vi "UpdateFilterMap.vi"(9 "MailBoxMessage":refnum<class "MailBoxMessage.lvclass">, 10 "_Msg-Filter":refnum<class "_Msg-Filter.lvclass">, 11 "MailboxClient in":refnum<class "MailboxClient.lvclass">) -> (3 "MailboxClient out":refnum<class "MailboxClient.lvclass">)   [LabVIEW 2020, in "MailboxClient.lvlib" / "MailboxClient.lvclass"]
uses:
  MailboxClient.lvclass
  <vilib>/Utility/miscctls.llb/LVMapReplaceAction.ctl
  MailboxManager/MailBoxMessage/MailBoxMessage.lvclass
  C:/Program Files (x86)/National Instruments/LabVIEW 2020/vi.lib/ActorFramework/Message/Message.lvclass
  C:/Users/taylo/Projects/LabVIEW/ActorMailbox/MailboxManager/MailBoxMessage/MailBoxMessage.lvclass
  MailboxManager/_Msg-Filter/_Msg-Filter.lvclass
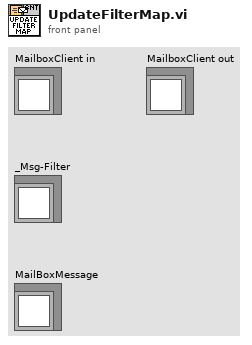
[diagram p1: front panel]
types:
  T1 = typedef "LVMapReplaceAction.ctl" = enum32{"Modify Entry only if found", "Add or Modify Entry", "Delete Entry"}
  T2 = map{refnum<class "Message.lvclass">, refnum<class "_Msg-Filter.lvclass">}
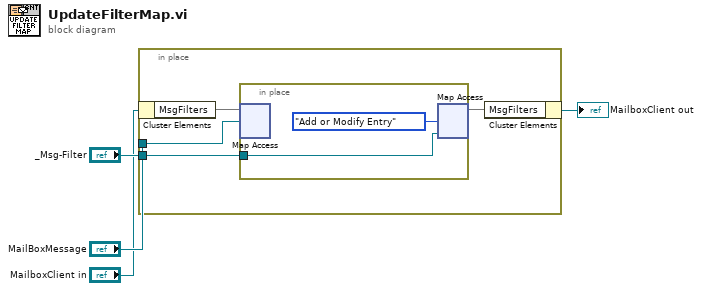
[diagram p0: block diagram]
diagram:
  n1 = in-place {
    in-place-border: "MailBoxMessage" -> [w6]
    in-place-border: "_Msg-Filter" -> [w5]
    n2 = in-place-cluster #1("MailboxClient in") -> ("MsgFilters"=w7:T2)
    n3 = in-place {
      in-place-border: w5 -> [w10]
      n4 = in-place-map #2(w7, w6) -> ()  [unwired: 1 in, 2 out]
      n5 = in-place-map #2(w10, LVMapReplaceAction."Add or Modify Entry" ("action")) -> (w8:T2)  [unwired: 2 out]
    }
    n6 = in-place-cluster #1("MsgFilters"=w8) -> (→"MailboxClient out":refnum<class "MailboxClient.lvclass">)
  }
